vi "ABXY Buttons.vi"(0 "Button Array":bool[](array[boolean])) -> (1 "A":T1(ring), 2 "B":T1(ring), 3 "X":T1(ring), 4 "Y":T1(ring))   [LabVIEW 2015]
doc: "This VI makes it easier to respond to A, B, X, Y button presses by providing states for each button press. There are four possible states for each button: Not Pressed, Pressed, Down, and Released."
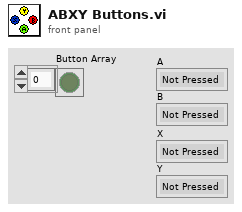
[diagram p1: front panel]
types:
  T1 = enum16{"Not Pressed", "Pressed", "Down", "Released"}
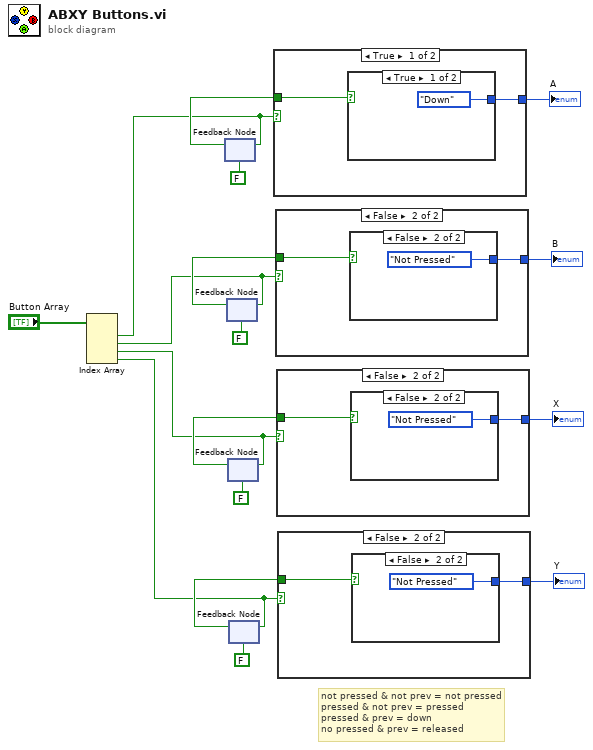
[diagram p0: block diagram]
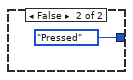
[diagram p2: hidden frame]
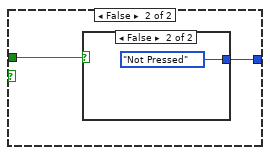
[diagram p3: hidden frame]
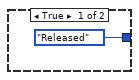
[diagram p4: hidden frame]
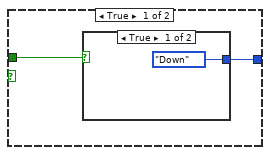
[diagram p5: hidden frame]
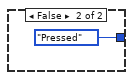
[diagram p6: hidden frame]
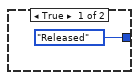
[diagram p7: hidden frame]
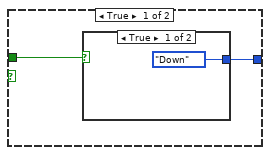
[diagram p8: hidden frame]
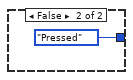
[diagram p9: hidden frame]
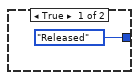
[diagram p10: hidden frame]
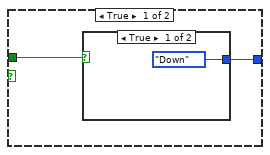
[diagram p11: hidden frame]
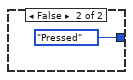
[diagram p12: hidden frame]
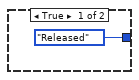
[diagram p13: hidden frame]
diagram:
  # "not pressed & not prev = not pressed\npressed & not prev = pressed\npressed & prev = down\nno pressed & prev = released"
  n1 = Index Array(array="Button Array") -> (element #1=w1:bool, element #2=w5:bool, element #3=w9:bool, element #4=w14:bool)  [unwired: 4 in]
  n2 = feedback #1(FALSE) -> (w3:bool)
  n3 = feedback-in #1(w1) -> ()
  n4 = feedback #2(FALSE) -> (w7:bool)
  n5 = feedback-in #2(w5) -> ()
  n6 = feedback #3(FALSE) -> (w11:bool)
  n7 = feedback-in #3(w9) -> ()
  n8 = feedback-in #4(w14) -> ()
  n9 = feedback #4(FALSE) -> (w15:bool)
  n10 = case shown="True" w1 {
    tunnel: w3 -> [w19 w23]
    tunnel: [w18 w22] -> w2
    frame True {
      n11 = case shown="True" w19 {
        tunnel: [T1."Down" ("Button") T1."Pressed" ("Button")] -> w18
        frame True {
        }
        frame False {
        }
      }
    }
    frame False {
      n12 = case shown="False" w23 {
        tunnel: [T1."Released" ("Button") T1."Not Pressed" ("Button")] -> w22
        frame True {
        }
        frame False {
        }
      }
    }
  }
  "A" <- w2
  n13 = case shown="False" w5 {
    tunnel: w7 -> [w27 w31]
    tunnel: [w26 w30] -> w6
    frame True {
      n14 = case shown="True" w27 {
        tunnel: [T1."Down" ("Button") T1."Pressed" ("Button")] -> w26
        frame True {
        }
        frame False {
        }
      }
    }
    frame False {
      n15 = case shown="False" w31 {
        tunnel: [T1."Released" ("Button") T1."Not Pressed" ("Button")] -> w30
        frame True {
        }
        frame False {
        }
      }
    }
  }
  "B" <- w6
  n16 = case shown="False" w9 {
    tunnel: w11 -> [w35 w39]
    tunnel: [w34 w38] -> w10
    frame True {
      n17 = case shown="True" w35 {
        tunnel: [T1."Down" ("Button") T1."Pressed" ("Button")] -> w34
        frame True {
        }
        frame False {
        }
      }
    }
    frame False {
      n18 = case shown="False" w39 {
        tunnel: [T1."Released" ("Button") T1."Not Pressed" ("Button")] -> w38
        frame True {
        }
        frame False {
        }
      }
    }
  }
  "X" <- w10
  n19 = case shown="False" w14 {
    tunnel: w15 -> [w43 w47]
    tunnel: [w42 w46] -> w13
    frame True {
      n20 = case shown="True" w43 {
        tunnel: [T1."Down" ("Button") T1."Pressed" ("Button")] -> w42
        frame True {
        }
        frame False {
        }
      }
    }
    frame False {
      n21 = case shown="False" w47 {
        tunnel: [T1."Released" ("Button") T1."Not Pressed" ("Button")] -> w46
        frame True {
        }
        frame False {
        }
      }
    }
  }
  "Y" <- w13
